vi "ICR_Hardware_Reset.vi"(8 "error in (no error)":errorcluster, 11 "HARDWARE Resources":T1={"AO6711 Physical Channels"="AnalogOutput/ao0:3", "AWG5421 Resource Name"="WaveformGenerator", "DIGIT 5122 Resource Name"="Digitizer", "HSDIO Resource Name"="SequencerHSDIO"}) -> (0 "error out":errorcluster)   [LabVIEW 2015]
doc: "This VI inits a waveform generation session for HSDIO 6541. This is a basic example that shows how to setup the board in order to generate waveforms according to a script. \n\n1. Initialize for a generation session.\n2. Assign specified channels in Channel List for dynamic operation : all = \"\" (default)\n3. Sets the Idle State for when the generation has completed : NO !!\n4. Configure the Sample clock to use the onboard clock, and configure the clock rate.\n5. Set generation mode to Scripted.\n6. Configure the Script Trigger : change to Digital Edge if waiting for an external\n trigger, and link Rising Edge and source trigger commands.\n Use PFI0 with SMB wired to the board, or any PFIxx if connected to accessory."
uses:
  controls/HARDWARE_Resources.ctl
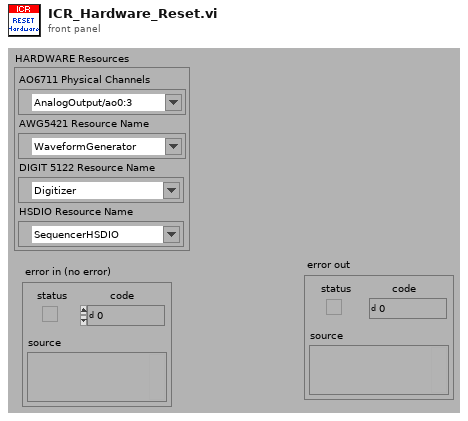
[diagram p1: front panel]
types:
  T1 = typedef "HARDWARE_Resources.ctl" = cluster{"AO6711 Physical Channels":tag, "AWG5421 Resource Name":refnum<k15>, "DIGIT 5122 Resource Name":refnum<k15>, "HSDIO Resource Name":refnum<k15>}
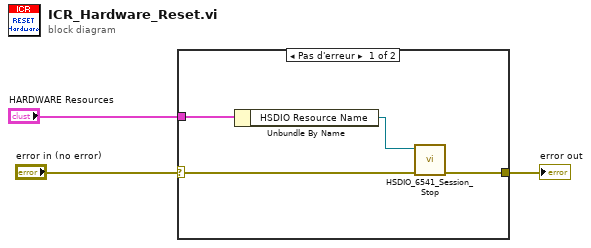
[diagram p0: block diagram]
diagram:
  n1 = case shown="Pas d'erreur" "error in (no error)" {
    selector: "error in (no error)" -> [w5 w8]
    tunnel: [w7 w8] -> w3
    tunnel: "HARDWARE Resources" -> [w4 _]
    frame No Error {
      n2 = Unbundle By Name(w4) -> ("HSDIO Resource Name"=w6:refnum<k15>)
      n3 = call "HSDIO_6541_Session_Stop.vi"("error in (no error)"=w5, "instrument handle in"=w6) -> ("error out"=w7:errorcluster)  [unwired: 9 in]
    }
    frame Error {
    }
  }
  "error out" <- w3
